vi "S4GUI.vi"(7 "Tab ObsEng":enum32{"Obs", "CCD modes", "Guider", "Eng"}(tab)) -> ()   [LabVIEW 2018] (continued)
      n64 = property on="Project ID" class="Str"(error in=w86, "Value"="" ("Observer"), "Text.BGColor"=u32 16448250) -> ()  [unwired: 1 in, 2 out]
      n65 = property on="SendExpose" class="Bool (strict)"(error in=w86, "Value"=TRUE ("ExtSync")) -> ()  [unwired: 1 in, 2 out]
      n66 = property on="suffix alert" class="Str"(error in=w86, "Text.BGColor"=u32 16711680, "Text.TextColor"=u32 16776722) -> ()  [unwired: 1 in, 2 out]
      n67 = property on="Object_dflat" class="Str"(error in=w86, "DisabledEnum"=w95) -> ()  [unwired: 1 in, 2 out]
      n68 = property on="Object_zero" class="Str"(error in=w86, "DisabledEnum"=w95) -> ()  [unwired: 1 in, 2 out]
      n69 = property on="Object_sflat" class="Str"(error in=w86, "DisabledEnum"=w95) -> ()  [unwired: 1 in, 2 out]
      n70 = local write "GUIDER"(FALSE ("GUIDER")) -> ()
      n71 = property on="Exptime ch1" class="DigNum (strict)"("Value"=w72) -> ()  [unwired: 2 in, 2 out]
      n72 = property on="Exptime ch2" class="DigNum (strict)"("Value"=w72) -> ()  [unwired: 2 in, 2 out]
      n73 = property on="Exptime ch3" class="DigNum (strict)"("Value"=w72) -> ()  [unwired: 2 in, 2 out]
      n74 = property on="Exptime ch4" class="DigNum (strict)"("Value"=w72) -> ()  [unwired: 2 in, 2 out]
      n75 = property on="dark suffix" class="Str"(error in=w82, "Text.BGColor"=u32 16448250) -> ()  [unwired: 1 in, 2 out]
      n76 = property on="object suffix" class="Str"(error in=w82, "Text.BGColor"=u32 16448250) -> (error out=w76:errorcluster)  [unwired: 1 in, 1 out]
      n77 = property on="dflat suffix" class="Str"(error in=w82, "Text.BGColor"=u32 16448250) -> ()  [unwired: 1 in, 2 out]
      n78 = property on="SET Temp message" class="Bool (strict)"(error in=w76, "Value"=TRUE ("SET Temp message")) -> (error out=w71:errorcluster)  [unwired: 1 in, 1 out]
      n79 = local write "TEST Comments"("Acquisition for testing purposes" ("TEST Comments")) -> ()
      n80 = local write "test suffix"("test" ("test suffix")) -> ()
      n81 = local write "Object_test"("TEST OBJECT" ("Object_test")) -> ()
      n82 = property on="sflat suffix" class="Str"(error in=w76, "Text.BGColor"=u32 16448250) -> ()  [unwired: 1 in, 2 out]
      n83 = property on="zero suffix" class="Str"(error in=w76, "Text.BGColor"=u32 16448250) -> ()  [unwired: 1 in, 2 out]
      n84 = property on="focus suffix" class="Str"(error in=w76, "Text.BGColor"=u32 16448250) -> ()  [unwired: 1 in, 2 out]
      "suffix alert" <- "Invalid char!" ("suffix alert")
      "FT warning" <- "" ("FT warning")
    }
    frame #4 {
      w97 = u32 1 ("# Cycles")
      n85 = local write "# Cycles"(w97) -> ()
      n86 = local write "#cycles ch1"(w97) -> ()
      n87 = local write "#cycles ch2"(w97) -> ()
      n88 = local write "#cycles ch3"(w97) -> ()
      n89 = local write "#cycles ch4"(w97) -> ()
      n90 = local write "Exp ch1"(w97) -> ()
      n91 = local write "Exp ch2"(w97) -> ()
      n92 = local write "Exp ch3"(w97) -> ()
      n93 = local write "Exp ch4"(w97) -> ()
    }
  }
  n94 = disable-structure shown="Enabled" {
    disable-tunnel: "S4ACS_GUI.lvclass" -> [w106 w108]
    disable-tunnel: w5 -> [w105 w107]
    disable-tunnel: [w100 w108] -> w25
    disable-tunnel: [w99 w107] -> w24
    frame Enabled {
      # "Carrega o ultimo filtro escolhido para os 4 canais."
      n95 = local read "Filter1"() -> (w104:u8)
      n96 = local read "Filter2"() -> (w103:u8)
      n97 = local read "Filter3"() -> (w102:u8)
      n98 = local read "Filter4"() -> (w101:u8)
      n99 = call-dynamic "LoadFilters.vi"("Filter 4"=w101, "Filter 3"=w102, "error in (no error)"=w105, "Filter 2"=w103, "Filter 1"=w104, "S4GUI in"=w106) -> ("error out"=w99:errorcluster, "S4GUI out"=w100:refnum<class "S4GUI.lvclass">)  [unwired: 4 in]
    }
    frame Disabled {
    }
  }
  n100 = flat-sequence "Indicadores dos canais da parte inferior da tela principal" {
    frame #0 {
      w109 = ""
      "B1" <- w109
      "PA1" <- w109
      "RO1" <- w109
      "G1" <- w109
      "SI2" <- w109
      "PA2" <- w109
      "G2" <- w109
      "B2" <- w109
      "RO2" <- w109
      "EA2" <- w109
      "SI3" <- w109
      "EA3" <- w109
      "PA3" <- w109
      "B3" <- w109
      "G3" <- w109
      "RO3" <- w109
      "SI4" <- w109
      "EA4" <- w109
      "PA4" <- w109
      "B4" <- w109
      "G4" <- w109
      "RO4" <- w109
      "SI1" <- w109
      "EA1" <- w109
    }
  }
  n101 = call-dynamic "Write GUI version.vi"("error in (no error)"=w24, "GUI version"=w22, "S4GUI in"=w25) -> ("error out"=w16:errorcluster, "S4GUI out"=w23:refnum<class "S4GUI.lvclass">)  [unwired: 7 in]
  n102 = property on="Tab Acq Type" class="TabCtl (strict)"(error in=w16, "DisabledEnum"=T12."Disabled and Grayed Out" ("Disabled")) -> (error out=w15:errorcluster)  [unwired: 1 in, 1 out]
  n103 = control-ref of="Current Configuration"() -> (w33:refnum<vi>)
  n104 = control-ref of="Parameters"() -> (w30:refnum<vi>)
  n105 = call-dynamic "Initialize.vi"("error in (no error)"=w15, "S4ACS_GUI in"=w23) -> ("error out"=w14:errorcluster, "S4ACS_GUI out"=w18:refnum<class "S4GUI.lvclass">)  [unwired: 8 in]
  n106 = property on="Tab Acq Type" class="TabCtl (strict)"(error in=w14, "DisabledEnum"=T12."Enabled" ("Disabled")) -> (error out=w13:errorcluster)  [unwired: 1 in, 1 out]
  n107 = property on="Property Node" class="Clust (strict)"(reference=w30, "Top"=230 ("Position:Top")) -> (reference out=w34:refnum<vi>)  [unwired: 1 in, 1 out]
  n108 = property on="Property Node" class="Clust (strict)"(reference=w33, "Top"=230 ("Position:Top")) -> (reference out=w32:refnum<vi>)  [unwired: 1 in, 1 out]
  n109 = call-dynamic "Read TabAcqType index.vi"("error in (no error)"=w13, "S4GUI in"=w18) -> ("error out"=w10:errorcluster, "TabAcqType index"=w17:u32, "S4GUI out"=w11:refnum<class "S4GUI.lvclass">)  [unwired: 7 in]
  n110 = case shown="1" w17 {
    tunnel: [T1."OBJECT" ("Tab Acq Type") T1."TEST" ("Tab Acq Type") T1."DFLAT" ("Tab Acq Type") T1."SFLAT" ("Tab Acq Type") T1."DARK" ("Tab Acq Type") T1."ZERO" ("Tab Acq Type") T1."FOCUS" ("Tab Acq Type")] -> w7
    frame 0, Default {
    }
    frame 1 {
    }
    frame 2 {
    }
    frame 3 {
    }
    frame 4 {
    }
    frame 5 {
    }
    frame 6 {
    }
  }
  n111 = local write "Tab Acq Type"(w7) -> ()
  n112 = Bundle("Parameters"=w34, "Current Configuration"=w32) -> (w31:T13)  [unwired: 1 in]
  n113 = call-dynamic "Write ExpMode.vi"("error in (no error)"=w10, "ExpMode"=w7, "S4GUI in"=w11) -> ("error out"=w9:errorcluster, "S4GUI out"=w8:refnum<class "S4GUI.lvclass">)  [unwired: 7 in]
  n114 = while {
    shift-right: [w135] -> w4
    shift-left: w8 -> [w137]
    shift-right: [w122] -> w2
    shift-left: w9 -> [w118]
    tunnel: w31 -> [w142]
    i -> [w128]
    stop <- w119 stop-if-true
    # "Sufixo do arquivo SEMPRE\nem minúsculas."
    n115 = case shown="\"TEST\"" "Tab Acq Type" {
      tunnel: ["object suffix" "test suffix" "dflat suffix" "sflat suffix" "dark suffix" "zero suffix" "focus suffix"] -> w130
      tunnel: ["OBJECT Comments" "TEST Comments" "DFLAT Comments" "SFLAT Comments" "DARK Comments" "ZERO Comments" "FOCUS Comments"] -> w143
      tunnel: ["OBJECT" "TEST" "FLAT" "FLAT" "DARK" "ZERO" "FOCUS"] -> w140
      tunnel: ["Object_obj" "Object_test" "DOMEFLAT" "SKYFLAT" "Object_dark" "ZERO" "Object_focus"] -> w139
      tunnel: [_ _ _ _ _ _ "Start focus"] -> w127
      tunnel: [_ _ _ _ _ _ "Step focus"] -> w125
      tunnel: [_ _ _ _ _ _ "#steps"] -> w126
      frame "OBJECT", Default {
      }
      frame "TEST" {
      }
      frame "DFLAT" {
      }
      frame "SFLAT" {
      }
      frame "DARK" {
      }
      frame "ZERO" {
      }
      frame "FOCUS" {
      }
    }
    n116 = flat-sequence {
      tunnel: w137 -> [w157]
      tunnel: [w157] -> w117
      tunnel: [w156] -> w134
      frame #0 {
        n117 = case shown="False" "reset max" {
          frame False {
          }
          frame True {
            n118 = local write "loop max(ms)"(u32 0 ("loop max(ms)")) -> ()
          }
        }
        n119 = Tick Count (ms)() -> (millisecond timer value=w156:u32)
      }
    }
    n120 = To Lower Case(string=w130) -> (all lower case string=w129:string)
    n121 = event shown="[44] \"Tab Acq Type\": Value Change" {
      selector: _ -> [_ _ _ _ _ _ _ _ _ _ _ _ _ _ _ _ _ _ _ _ _ _ _ _ _ _ _ _ _ _ _ _ _ _ _ _ _ _ _ _ _ _ _ _ _ _ _ _ _ _ _ _ _ _ _ _ _ _ _ _ _ _ _ _ _ _ _ _ _ _ _ _ _ _ _ _ _ _ _ _ _ _ _ _ _ _ _ _ _ _ _ _ _ _ _ _ _ _ _ _ _ _ _ _ _ _ _ _ _ _ _ _ _ _ _ _ _ _ _ _ _ _ _ _ _ _ _ _ _ _ _ _ _ _ _ _ _ _ _ _ _ _ _ _ _]
      dyn-events: _ -> [_ _ _ _ _ _ _ _ _ _ _ _ _ _ _ _ _ _ _ _ _ _ _ _ _ _ _ _ _ _ _ _ _ _ _ _ _ _ _ _ _ _ _ _ _ _ _ _ _ _ _ _ _ _ _ _ _ _ _ _ _ _ _ _ _ _ _ _ _ _ _ _ _ _ _ _ _ _ _ _ _ _ _ _ _ _ _ _ _ _ _ _ _ _ _ _ _ _ _ _ _ _ _ _ _ _ _ _ _ _ _ _ _ _ _ _ _ _ _ _ _ _ _ _ _ _ _ _ _ _ _ _ _ _ _ _ _ _ _ _ _ _ _ _ _]
      timeout: 20 -> [_ _ _ _ _ _ _ _ _ _ _ _ _ _ _ _ _ _ _ _ _ _ _ _ _ _ _ _ _ _ _ _ _ _ _ _ _ _ _ _ _ _ _ _ _ _ _ _ _ _ _ _ _ _ _ _ _ _ _ _ _ _ _ _ _ _ _ _ _ _ _ _ _ _ _ _ _ _ _ _ _ _ _ _ _ _ _ _ _ _ _ _ _ _ _ _ _ _ _ _ _ _ _ _ _ _ _ _ _ _ _ _ _ _ _ _ _ _ _ _ _ _ _ _ _ _ _ _ _ _ _ _ _ _ _ _ _ _ _ _ _ _ _ _ _]
      tunnel: w117 -> [w199 w2003 w2014 w2019 w2024 w2029 w2034 w2039 w2357 w2516 w2546 w2552 w2574 w2596 w2795 w2803 w2882 w2903 w2975 w3046 w3147 w3161 w3302 w3541 w3573 w3605 w3637 w3672 w3707 w3742 w3777 w3780 w3878 w4087 w4151 w4678 w4757 w4829 w4900 w4973 w5024 w5065 w5507 w5513 w5633 w7076 w7220 w7425 w7613 w7877 w8136 w8151 w8362 w8592 w8616 w8640 w8664 w8688 w8703 w8845 w8987 w9116 w9136 w9156 w9176 w9197 w9262 w9327 w9392 w9457 w9494 w9522 w9550 w9579 w9652 w9782 w9816 w9875 w9934 w9993 w10052 w10072 w10099 w10115 w10136 w10166 w10196 w10221 w10262 w10303 w10344 w10385 w10426 w10467 w10508 w10551 w10666 w10776 w10886 w10995 w11005 w11025 w11040 w11055 w11070 w11085 w11100 w11115 w11130 w11161 w11190 w11214 w11256 w11290 w11317 w11340 w11368 w11388 w11403 w11423 w11506 w11834 w11860 w12026 w12046 w12061 w12077 w12097 w12117 w12137 w12157 w12172 w12188 w12208 w12228 w12248 w12268 w12283 w12303 w12323 w12343 w12358 w12378 w12398 w12418]
      tunnel: w118 -> [w198 w2002 w2013 w2018 w2023 w2028 w2033 w2038 w2358 w2514 w2545 w2551 w2573 w2595 w2794 w2802 w2881 w2902 w2974 w3047 w3146 w3153 w3298 w3540 w3572 w3604 w3636 w3671 w3706 w3741 w3776 w3788 w3879 w4086 w4150 w4677 w4756 w4828 w4896 w4972 w5022 w5064 w5463 w5512 w5632 w7075 w7219 w7424 w7612 w7870 w8134 w8150 w8360 w8591 w8615 w8639 w8663 w8687 w8702 w8843 w8986 w9117 w9137 w9157 w9177 w9196 w9261 w9326 w9391 w9455 w9492 w9520 w9548 w9578 w9651 w9781 w9815 w9874 w9933 w9992 w10051 w10071 w10098 w10114 w10135 w10165 w10195 w10220 w10261 w10302 w10343 w10384 w10425 w10466 w10507 w10550 w10665 w10775 w10885 w10994 w11004 w11024 w11039 w11054 w11069 w11084 w11099 w11114 w11129 w11160 w11189 w11213 w11255 w11289 w11316 w11339 w11367 w11387 w11402 w11422 w11507 w11833 w11859 w12025 w12045 w12060 w12076 w12096 w12116 w12136 w12156 w12171 w12187 w12207 w12227 w12247 w12267 w12282 w12302 w12322 w12342 w12357 w12377 w12397 w12417]
      tunnel: [w195 w2001 w2011 w2015 w2020 w2025 w2030 w2035 w2320 w2508 w2533 w2553 w2575 w2597 w2782 w2820 w2881 w2920 w2992 w3064 w3133 w3159 w3300 w3451 w3559 w3591 w3623 w3662 w3697 w3732 w3767 w3788 w3801 w4007 w4138 w4597 w4754 w4826 w4891 w4970 w5025 w5059 w5466 w5509 w5600 w7129 w7213 w7418 w7624 w7871 w8135 w8143 w8348 w8522 w8598 w8623 w8647 w8671 w8689 w8832 w8972 w9115 w9135 w9155 w9175 w9195 w9260 w9325 w9390 w9456 w9493 w9521 w9549 w9583 w9656 w9783 w9814 w9873 w9932 w9991 w10050 w10070 w10097 w10113 w10134 w10164 w10194 w10223 w10264 w10305 w10346 w10387 w10428 w10469 w10510 w10549 w10664 w10774 w10884 w10991 w11003 w11023 w11038 w11053 w11068 w11083 w11098 w11113 w11128 w11145 w11187 w11212 w11254 w11288 w11315 w11338 w11350 w11370 w11390 w11406 w11430 w11841 w11864 w12008 w12028 w12048 w12069 w12082 w12102 w12119 w12139 w12159 w12176 w12191 w12211 w12230 w12250 w12270 w12286 w12305 w12325 w12345 w12361 w12380 w12400] -> w122
      tunnel: [w196 _ _ _ _ _ _ _ _ _ _ _ _ _ _ _ _ _ _ _ _ _ _ _ _ _ _ _ _ _ _ _ _ _ _ _ _ _ _ _ _ _ _ _ _ _ _ _ _ _ _ _ _ _ _ _ _ _ _ _ _ _ _ _ _ _ _ _ _ _ _ _ _ _ _ _ _ _ _ _ _ _ _ _ _ _ _ _ _ _ _ _ _ _ _ _ _ _ _ _ _ _ _ _ _ _ _ _ _ _ _ _ _ _ _ _ _ _ _ _ _ _ _ _ _ _ _ _ _ _ _ _ _ _ _ _ _ _ _ _ _ _ _ _ _] -> w120
      tunnel: w129 -> [_ _ _ _ _ _ _ _ _ _ _ _ _ _ _ _ _ _ _ _ _ _ _ _ _ _ _ _ _ _ _ _ _ _ _ _ _ _ _ _ _ w5058 _ _ _ _ w7218 w7422 _ w7875 _ w8148 w8369 _ _ _ _ _ w8710 w8852 w8994 _ _ _ _ _ _ _ _ _ _ _ _ _ _ _ _ _ _ _ _ _ _ _ _ _ _ _ _ _ _ _ _ _ _ _ _ _ _ _ _ _ _ _ _ _ _ _ _ _ _ _ _ _ _ _ _ _ _ _ _ _ _ _ _ _ _ _ _ _ _ _ _ _ _ _ _ _ _ _ _ _ _ _ _]
      tunnel: w143 -> [_ _ _ _ _ _ _ _ _ _ _ _ _ _ _ _ _ _ _ _ _ _ _ _ _ _ _ _ _ _ _ _ _ _ _ _ _ _ _ _ _ w5057 _ _ _ _ w7217 _ w7628 w7874 _ w8147 w8368 _ _ _ _ _ w8709 w8851 w8993 _ _ _ _ _ _ _ _ _ _ _ _ _ _ _ _ _ _ _ _ _ _ _ _ _ _ _ _ _ _ _ _ _ _ _ _ _ _ _ _ _ _ _ _ _ _ _ _ _ _ _ _ _ _ _ _ _ _ _ _ _ _ _ _ _ _ _ _ _ _ _ _ _ _ _ _ _ _ _ _ _ _ _ _]
      tunnel: w142 -> [_ _ _ _ _ _ _ _ _ _ _ _ _ _ _ _ _ _ _ _ _ _ _ _ _ _ _ _ _ _ _ w3781 _ _ _ _ _ _ _ _ _ _ _ _ _ _ _ _ _ _ _ _ _ _ _ _ _ _ _ _ _ _ _ _ _ _ _ _ _ _ _ _ _ _ _ _ _ _ _ _ _ _ _ _ _ _ _ _ _ _ _ _ _ _ _ _ _ _ _ _ _ _ _ _ _ _ _ _ _ _ _ _ _ _ _ _ _ _ _ _ _ _ _ _ _ _ _ _ _ _ _ _ _ _ _ _ _ _ _ _ _ _ _ _ _]
      tunnel: [w194 w2003 w2012 w2016 w2021 w2026 w2031 w2036 w2322 w2507 w2534 w2554 w2576 w2598 w2783 w2821 w2882 w2921 w2993 w3065 w3124 w3160 w3301 w3453 w3550 w3582 w3614 w3639 w3674 w3709 w3744 w3780 w3802 w4004 w4139 w4598 w4755 w4827 w4892 w4971 w5026 w5039 w5467 w5508 w5601 w7128 w7214 w7419 w7625 w7872 w8136 w8144 w8349 w8523 w8599 w8624 w8648 w8672 w8690 w8831 w8974 w9114 w9134 w9154 w9174 w9194 w9259 w9324 w9389 w9454 w9491 w9519 w9547 w9581 w9654 w9784 w9813 w9872 w9931 w9990 w10049 w10069 w10089 w10112 w10133 w10163 w10193 w10222 w10263 w10304 w10345 w10386 w10427 w10468 w10509 w10548 w10663 w10773 w10883 w10992 w10996 w11019 w11034 w11049 w11064 w11079 w11094 w11109 w11124 w11144 w11162 w11199 w11223 w11271 w11301 w11326 w11349 w11369 w11389 w11404 w11431 w11842 w11865 w12007 w12027 w12047 w12068 w12080 w12100 w12118 w12138 w12158 w12175 w12189 w12209 w12229 w12249 w12269 w12284 w12304 w12324 w12344 w12359 w12379 w12399] -> w136
      tunnel: "Input Cluster" -> [_ _ _ _ _ _ _ _ _ _ _ _ _ _ _ _ _ _ _ _ _ _ _ _ _ _ _ _ _ _ _ w3779 _ _ _ _ _ _ _ _ _ _ _ _ _ _ _ _ _ _ _ _ _ _ _ _ _ _ _ _ _ _ _ _ _ _ _ _ _ _ _ _ _ _ _ _ _ _ _ _ _ _ _ _ _ _ _ _ _ _ _ _ _ _ _ _ _ _ _ _ _ _ _ _ _ _ _ _ _ _ _ _ _ _ _ _ _ _ _ _ _ _ _ _ _ _ _ _ _ _ _ _ _ _ _ _ _ _ _ _ _ _ _ _ _]
      tunnel: w140 -> [_ _ _ _ _ _ _ _ _ _ _ _ _ _ _ _ _ _ _ _ _ _ _ _ _ _ _ _ _ _ _ _ _ _ _ _ _ _ _ _ _ w5056 _ _ _ _ w7215 w7420 w7626 w7873 _ w8145 w8367 _ _ _ _ _ w8708 w8849 w8992 _ _ _ _ _ _ _ _ _ _ _ _ _ _ _ _ _ _ _ _ _ _ _ _ _ _ _ _ _ _ _ _ _ _ _ _ _ _ _ _ _ _ _ _ _ _ _ _ _ _ _ _ _ _ _ _ _ _ _ _ _ _ _ _ _ _ _ _ _ _ _ _ _ _ _ _ _ _ _ _ _ _ _ _]
      tunnel: w139 -> [_ _ _ _ _ _ _ _ _ _ _ _ _ _ _ _ _ _ _ _ _ _ _ _ _ _ _ _ _ _ _ _ _ _ _ _ _ _ _ _ _ w5055 _ _ _ _ _ w7423 w7629 w7876 _ w8149 w8366 _ _ _ _ _ w8707 w8850 w8991 _ _ _ _ _ _ _ _ _ _ _ _ _ _ _ _ _ _ _ _ _ _ _ _ _ _ _ _ _ _ _ _ _ _ _ _ _ _ _ _ _ _ _ _ _ _ _ _ _ _ _ _ _ _ _ _ _ _ _ _ _ _ _ _ _ _ _ _ _ _ _ _ _ _ _ _ _ _ _ _ _ _ _ _]
      tunnel: "Observer" -> [_ _ _ _ _ _ _ _ _ _ _ _ _ _ _ _ _ _ _ _ _ _ _ _ _ _ _ _ _ _ _ _ _ _ _ _ _ _ _ _ _ w5054 _ _ w5606 w6963 w7216 w7421 w7627 _ _ w8146 w8365 _ _ _ _ _ w8706 w8848 w8990 _ _ _ _ _ _ _ _ _ _ _ _ _ _ _ _ _ _ _ _ _ _ _ _ _ _ _ _ _ _ _ _ _ _ _ _ _ _ _ _ _ _ _ _ _ _ _ _ _ _ _ _ _ _ _ _ _ _ _ _ _ _ _ _ _ _ _ _ _ _ _ _ _ _ _ _ _ _ _ _ _ _ _ _]
      tunnel: w128 -> [w197 _ _ _ _ _ _ _ _ _ _ _ _ _ _ _ _ _ _ _ _ _ _ _ _ _ _ _ _ _ _ _ _ _ _ _ _ _ _ _ _ _ _ _ _ _ _ _ _ _ _ _ _ _ _ _ _ _ _ _ _ _ _ _ _ _ _ _ _ _ _ _ _ _ _ _ _ _ _ _ _ _ _ _ _ _ _ _ _ _ _ _ _ _ _ _ _ _ _ _ _ _ _ _ _ _ _ _ _ _ _ _ _ _ _ _ _ _ _ _ _ _ _ _ _ _ _ _ _ _ _ _ _ _ _ _ _ _ _ _ _ _ _ _ _]
      tunnel: "Tab Acq Type" -> [_ _ _ _ _ _ _ _ _ _ _ _ _ _ _ _ _ _ _ _ _ _ _ _ _ _ _ _ _ _ _ _ _ _ _ _ _ _ _ _ _ w5046 _ _ _ _ _ _ w7615 _ _ _ w8356 _ _ _ _ _ w8697 w8839 w8980 _ _ _ _ _ _ _ _ _ _ _ _ _ _ _ _ _ _ _ _ _ _ _ _ _ _ _ _ _ _ _ _ _ _ _ _ _ _ _ _ _ _ _ _ _ _ _ _ _ _ _ _ _ _ _ _ _ _ _ _ _ _ _ _ _ _ _ _ _ _ _ _ _ _ _ _ _ _ _ _ _ _ _ _]
      tunnel: w127 -> [_ _ _ _ _ _ _ _ _ _ _ _ _ _ _ _ _ _ _ _ _ _ _ _ _ _ _ _ _ _ _ _ _ _ _ _ _ _ _ _ _ w5045 _ _ _ _ _ _ _ _ _ _ w8355 _ _ _ _ _ w8696 w8838 w8979 _ _ _ _ _ _ _ _ _ _ _ _ _ _ _ _ _ _ _ _ _ _ _ _ _ _ _ _ _ _ _ _ _ _ _ _ _ _ _ _ _ _ _ _ _ _ _ _ _ _ _ _ _ _ _ _ _ _ _ _ _ _ _ _ _ _ _ _ _ _ _ _ _ _ _ _ _ _ _ _ _ _ _ _]
      tunnel: w126 -> [_ _ _ _ _ _ _ _ _ _ _ _ _ _ _ _ _ _ _ _ _ _ _ _ _ _ _ _ _ _ _ _ _ _ _ _ _ _ _ _ _ w5043 _ _ _ _ _ _ _ _ _ _ w8353 _ _ _ _ _ w8694 w8836 w8977 _ _ _ _ _ _ _ _ _ _ _ _ _ _ _ _ _ _ _ _ _ _ _ _ _ _ _ _ _ _ _ _ _ _ _ _ _ _ _ _ _ _ _ _ _ _ _ _ _ _ _ _ _ _ _ _ _ _ _ _ _ _ _ _ _ _ _ _ _ _ _ _ _ _ _ _ _ _ _ _ _ _ _ _]
      tunnel: w125 -> [_ _ _ _ _ _ _ _ _ _ _ _ _ _ _ _ _ _ _ _ _ _ _ _ _ _ _ _ _ _ _ _ _ _ _ _ _ _ _ _ _ w5044 _ _ _ _ _ _ _ _ _ _ w8354 _ _ _ _ _ w8695 w8837 w8978 _ _ _ _ _ _ _ _ _ _ _ _ _ _ _ _ _ _ _ _ _ _ _ _ _ _ _ _ _ _ _ _ _ _ _ _ _ _ _ _ _ _ _ _ _ _ _ _ _ _ _ _ _ _ _ _ _ _ _ _ _ _ _ _ _ _ _ _ _ _ _ _ _ _ _ _ _ _ _ _ _ _ _ _]
      tunnel: "Project ID" -> [_ _ _ _ _ _ _ _ _ _ _ _ _ _ _ _ _ _ _ _ _ _ _ _ _ _ _ _ _ _ _ _ _ _ _ _ _ _ _ _ _ _ _ _ w5605 w6961 _ _ _ _ _ _ _ _ _ _ _ _ _ _ _ _ _ _ _ _ _ _ _ _ _ _ _ _ _ _ _ _ _ _ _ _ _ _ _ _ _ _ _ _ _ _ _ _ _ _ _ _ _ _ _ _ _ _ _ _ _ _ _ _ _ _ _ _ _ _ _ _ _ _ _ _ _ _ _ _ _ _ _ _ _ _ _ _ _ _ _ _ _ _ _ _ _ _ _]
      event Timeout {
        # "execução do botão\nOK do SET TEMP de\ntodos os canais."
        # "2024.07.02: Mostra as publicações das aplicações."
        # "Trata as tarefas para atender \naos clientes: Publisher"
        # "Conteudo dos indicadores"
        # "Status dos indicadores: Habilitado ou Desab."
        # "Obtém os valores de status dos\ndispositivos de cada servidor para\napresentar nos indicadores da GUI."
        # "Trata as tarefas individuais de \ncada servidor (ACS1,...,ACS4, \nICS, TCS, Focus,Weather)"
        # "Determina a sequência de\ntarefas dos servidores\npara uma observação, de \nacordo com o modo de \noperação (disparado com \nos botões START)"
        # "execução dos botões\n no modo sincrono."
        # "execução dos botões\n no modo assincrono."
        n122 = event-data() -> ()  [unwired: 1 in, 2 out]
        n123 = disable-structure shown="Enabled" {
          disable-tunnel: w199 -> [w236 _]
          disable-tunnel: w198 -> [w234 _]
          frame Disabled {
            n124 = flat-sequence {
              tunnel: [w245] -> w235
              tunnel: w236 -> [w245]
              tunnel: w234 -> [w244]
              tunnel: [w244] -> w233
              frame #0 {
                n125 = local read "time alert"() -> (w242:u32)
                n126 = Tick Count (ms)() -> (millisecond timer value=w243:u32)
                n127 = Subtract(x=w243, y=w242) -> (x-y=w241:u32)
                n128 = Greater?(x=w241, y=u32 750) -> (0:w239:bool)
                n129 = case shown="True" w239 {
                  frame False {
                  }
                  frame True {
                    n130 = property on="suffix alert" class="Str"("Visible"=FALSE) -> ()  [unwired: 2 in, 2 out]
                  }
                }
              }
            }
            n131 = local read "charKeyboardInteger"() -> (w237:i16)
            n132 = call-dynamic "Read ExpMode.vi"("error in (no error)"=w233, "S4GUI in"=w235) -> ("ExpMode"=w238:T1)  [unwired: 7 in, 2 out]
            n133 = case shown="Default" w237 {
              tunnel: w238 -> [_ w247 w269]
              frame 32767 {
              }
              frame 0, 8, 32, 48..57, 65..90, 97..122 {
                n134 = case shown="\"OBJECT\", Default" w247 {
                  tunnel: [w252 w253 w254 w255 w256 w257] -> w248
                  frame "OBJECT", Default {
                    n135 = local read "object suffix"() -> (w252:string)
                  }
                  frame "DFLAT" {
                    n136 = local read "dflat suffix"() -> (w253:string)
                  }
                  frame "SFLAT" {
                    n137 = local read "sflat suffix"() -> (w254:string)
                  }
                  frame "DARK" {
                    n138 = local read "dark suffix"() -> (w255:string)
                  }
                  frame "ZERO" {
                    n139 = local read "zero suffix"() -> (w256:string)
                  }
                  frame "FOCUS" {
                    n140 = local read "focus suffix"() -> (w257:string)
                  }
                }
                n141 = String Length(string=w248) -> (length=w251:i32)
                n142 = Greater?(x=w251, y=10) -> (0:w249:bool)
                n143 = case shown="True" w249 {
                  tunnel: w248 -> [w258 _]
                  tunnel: w247 -> [_ w260]
                  frame False {
                    n144 = local write "suffix temp"(w258) -> ()
                  }
                  frame True {
                    n145 = local read "suffix temp"() -> (w259:string)
                    n146 = case shown="\"OBJECT\", Default" w260 {
                      tunnel: w259 -> [w261 w262 w263 w264 w265 w266]
                      frame "OBJECT", Default {
                        n147 = local write "object suffix"(w261) -> ()
                      }
                      frame "DFLAT" {
                        n148 = local write "dflat suffix"(w262) -> ()
                      }
                      frame "SFLAT" {
                        n149 = local write "sflat suffix"(w263) -> ()
                      }
                      frame "DARK" {
                        n150 = local write "dark suffix"(w264) -> ()
                      }
                      frame "ZERO" {
                        n151 = local write "zero suffix"(w265) -> ()
                      }
                      frame "FOCUS" {
                        n152 = local write "focus suffix"(w266) -> ()
                      }
                    }
                  }
                }
              }
              frame Default {
                n153 = local write "charKeyboardInteger"(i16 32767 ("lastChar")) -> ()
                n154 = Tick Count (ms)() -> (millisecond timer value=→"time alert":u32)
                n155 = property on="suffix alert" class="Str"("Visible"=TRUE) -> ()  [unwired: 2 in, 2 out]
                n156 = case shown="\"OBJECT\", Default" w269 {
                  tunnel: "suffix temp" -> [w272 w273 w274 w275 w276 w277]
                  frame "OBJECT", Default {
                    n157 = local write "object suffix"(w272) -> ()
                  }
                  frame "DFLAT" {
                    n158 = local write "dflat suffix"(w273) -> ()
                  }
                  frame "SFLAT" {
                    n159 = local write "sflat suffix"(w274) -> ()
                  }
                  frame "DARK" {
                    n160 = local write "dark suffix"(w275) -> ()
                  }
                  frame "ZERO" {
                    n161 = local write "zero suffix"(w276) -> ()
                  }
                  frame "FOCUS" {
                    n162 = local write "focus suffix"(w277) -> ()
                  }
                }
              }
            }
          }
          frame Enabled {
          }
        }
        n163 = disable-structure shown="Enabled" {
          disable-tunnel: w199 -> [w283 w288]
          disable-tunnel: w198 -> [w282 w286]
          disable-tunnel: [w280 w285] -> w191
          disable-tunnel: [w279 w284] -> w193
          disable-tunnel: w197 -> [_ w287]
          frame Disabled {
            n164 = call "Elapsed Time"() -> ("Time has Elapsed"=w278:bool)  [unwired: 12 in, 7 out]
            n165 = call "Elapsed Time3"() -> ("Time has Elapsed"=w281:bool)  [unwired: 12 in, 7 out]
            n166 = call "Write Status_timeout.vi"("error in (no error)"=w282, "TCS_timeout"=w281, "Status_timeout"=w278, "S4ACS_GUI in"=w283) -> ("error out"=w280:errorcluster, "S4ACS_GUI out"=w279:refnum<class "S4GUI.lvclass">)  [unwired: 6 in]
          }
          frame Enabled {
            n167 = call-dynamic "Write loop counter.vi"("error in (no error)"=w286, "loop counter"=w287, "S4GUI in"=w288) -> ("error out"=w285:errorcluster, "S4GUI out"=w284:refnum<class "S4GUI.lvclass">)  [unwired: 7 in]
          }
        }
        n168 = call-dynamic "HandleSetTemp.vi"("error in (no error)"=w191, "S4GUI in"=w193) -> ("error out"=w190:errorcluster, "S4GUI out"=w192:refnum<class "S4GUI.lvclass">)  [unwired: 8 in]
        n169 = call-dynamic "GetPubs.vi"("error in (no error)"=w190, "S4GUI in"=w192) -> ("error out"=w210:errorcluster, "Pubs out"=→"All Pubs":T11, "S4GUI out"=w209:refnum<class "S4GUI.lvclass">)  [unwired: 7 in]
        n170 = call-dynamic "HandlePauseAsync.vi"("error in (no error)"=w210, "S4GUI in"=w209) -> ("error out"=w227:errorcluster, "S4GUI out"=w229:refnum<class "S4GUI.lvclass">)  [unwired: 8 in]
        n171 = call-dynamic "HandleStopAsync.vi"("error in (no error)"=w227, "S4GUI in"=w229) -> ("error out"=w226:errorcluster, "S4GUI out"=w228:refnum<class "S4GUI.lvclass">)  [unwired: 8 in]
        n172 = call-dynamic "HandleAbortAsync.vi"("error in (no error)"=w226, "S4GUI in"=w228) -> ("error out"=w220:errorcluster, "S4GUI out"=w221:refnum<class "S4GUI.lvclass">)  [unwired: 8 in]
        n173 = call-dynamic "HandlePauseSync.vi"("error in (no error)"=w220, "S4GUI in"=w221) -> ("error out"=w219:errorcluster, "S4GUI out"=w218:refnum<class "S4GUI.lvclass">)  [unwired: 8 in]
        n174 = call-dynamic "HandleStopSync.vi"("error in (no error)"=w219, "S4GUI in"=w218) -> ("error out"=w223:errorcluster, "S4GUI out"=w225:refnum<class "S4GUI.lvclass">)  [unwired: 8 in]
        n175 = call-dynamic "HandleAbortSync.vi"("error in (no error)"=w223, "S4GUI in"=w225) -> ("error out"=w222:errorcluster, "S4GUI out"=w224:refnum<class "S4GUI.lvclass">)  [unwired: 8 in]
        n176 = call-dynamic "HandleObservation.vi"("error in (no error)"=w222, "S4ACS_GUI in"=w224) -> ("error out"=w231:errorcluster, "S4ACS_GUI out"=w232:refnum<class "S4GUI.lvclass">)  [unwired: 8 in]
        n177 = call-dynamic "HandleServers.vi"("error in (no error)"=w231, "S4GUI in"=w232) -> ("error out"=w213:errorcluster, "S4GUI out"=w214:refnum<class "S4GUI.lvclass">)  [unwired: 8 in]
        n178 = call-dynamic "HandleClients.vi"("error in (no error)"=w213, "S4GUI in"=w214) -> ("error out"=w212:errorcluster, "S4GUI out"=w204:refnum<class "S4GUI.lvclass">)  [unwired: 8 in]
        n179 = call-dynamic "GetStatus.vi"("error in (no error)"=w212, "S4GUI in"=w204) -> ("error out"=w206:errorcluster, "S4GUI out"=w203:refnum<class "S4GUI.lvclass">)  [unwired: 8 in]
        n180 = call-dynamic "Read output cluster.vi"("error in (no error)"=w206, "S4GUI in"=w203) -> ("error out"=w205:errorcluster, "output cluster"=w200:T15, "S4GUI out"=w202:refnum<class "S4GUI.lvclass">)  [unwired: 7 in]
        n181 = call "Elapsed Time2"() -> ("Time has Elapsed"=w217:bool)  [unwired: 12 in, 7 out]
        n182 = call-dynamic "Read Cluster Disable.vi"("error in (no error)"=w205, "S4GUI in"=w202) -> ("error out"=w207:errorcluster, "Cluster Disable"=w208:T16, "S4GUI out"=w201:refnum<class "S4GUI.lvclass">)  [unwired: 7 in]
        n183 = call "Read cfg file.vi"("error in (no error)"=w207, "S4ACS_GUI in"=w201) -> ("error out"=w215:errorcluster, "cfg file"=w230:string, "S4ACS_GUI out"=w216:refnum<class "S4GUI.lvclass">)  [unwired: 7 in]
        n184 = case shown="True" w217 {
          tunnel: w200 -> [_ w346]
          tunnel: w208 -> [_ w345]
          tunnel: w230 -> [_ w344]
          tunnel: w216 -> [w291 w343]
          tunnel: w215 -> [w290 w342]
          tunnel: [w290 w295] -> w195
          tunnel: [FALSE ("exit") w294] -> w196
          tunnel: [w291 w293] -> w194
          frame False {
          }
          frame True {
            w302 = "arking" ("regular expression")
            w320 = "ERRO" ("regular expression")
            # "Verifica mudança de modo e se deve carregar valores default \npara procedimento de ajuste de foco do telescópio."
            # "1a vez FOTOM (F)"
            # "1a vez POLAR (F)"
            # "MODE:\nF -> photometric\nT -> polarimetric"
            n185 = stacked-sequence {
              tunnel: w343 -> [w395 w402 w413 w423 w432]
              tunnel: w342 -> [w394 w401 w412 w422 w431]
              tunnel: [_ _ _ _ w430] -> w336
              tunnel: [_ _ _ _ w429] -> w335
              tunnel: [_ _ _ _ w428] -> w305
              frame #0 {
                n186 = call-dynamic "Read AcquisitionA.vi"("error in (no error)"=w394, "S4ACS_GUI in"=w395) -> ("error out"=w391:errorcluster, "Acquisition.lvclass"=w393:refnum<class "Acquisition.lvclass">)  [unwired: 7 in, 1 out]
                n187 = call-dynamic "Read Channel.vi"("error in (no error)"=w391, "Acquisition in"=w393) -> ("error out"=w390:errorcluster, "Channel.lvclass"=w392:refnum<class "Channel.lvclass">)  [unwired: 7 in, 1 out]
                n188 = call-dynamic "Read CyclesDone.vi"("error in (no error)"=w390, "Channel in"=w392) -> ("error out"=→"error out 6":errorcluster, "CyclesDone"=w387:u32)  [unwired: 7 in, 1 out]
                "Cycles Done ch1" <- w387
                n189 = Number To Decimal String(number=w387) -> (decimal integer string=w386:string)  [unwired: 1 in]
                n190 = Concatenate Strings("#Cycles Done ", w386) -> (w385:string)
                n191 = property on="Cycles Done ch1" class="Slide (strict)"("Caption.Text"=w385) -> ()  [unwired: 2 in, 2 out]
              }
              frame #1 {
                n192 = call "Read AcquisitionB.vi"("error in (no error)"=w401, "S4ACS_GUI in"=w402) -> ("error out"=w404:errorcluster, "Acquisition.lvclass"=w405:refnum<class "Acquisition.lvclass">)  [unwired: 7 in, 1 out]
                n193 = call-dynamic "Read Channel.vi"("error in (no error)"=w404, "Acquisition in"=w405) -> ("error out"=w403:errorcluster, "Channel.lvclass"=w406:refnum<class "Channel.lvclass">)  [unwired: 7 in, 1 out]
                n194 = call-dynamic "Read CyclesDone.vi"("error in (no error)"=w403, "Channel in"=w406) -> ("error out"=→"error out 4":errorcluster, "CyclesDone"=w397:u32)  [unwired: 7 in, 1 out]
                "Cycles Done ch2" <- w397
                n195 = Number To Decimal String(number=w397) -> (decimal integer string=w398:string)  [unwired: 1 in]
                n196 = Concatenate Strings("#Cycles Done ", w398) -> (w396:string)
                n197 = property on="Cycles Done ch2" class="Slide (strict)"("Caption.Text"=w396) -> ()  [unwired: 2 in, 2 out]
              }
              frame #2 {
                n198 = call-dynamic "Read AcquisitionC.vi"("error in (no error)"=w412, "S4ACS_GUI in"=w413) -> ("error out"=w415:errorcluster, "Acquisition.lvclass"=w416:refnum<class "Acquisition.lvclass">)  [unwired: 7 in, 1 out]
                n199 = call-dynamic "Read Channel.vi"("error in (no error)"=w415, "Acquisition in"=w416) -> ("error out"=w414:errorcluster, "Channel.lvclass"=w417:refnum<class "Channel.lvclass">)  [unwired: 7 in, 1 out]
                n200 = call-dynamic "Read CyclesDone.vi"("error in (no error)"=w414, "Channel in"=w417) -> ("error out"=→"error out 5":errorcluster, "CyclesDone"=w408:u32)  [unwired: 7 in, 1 out]
                "Cycles Done ch3" <- w408
                n201 = Number To Decimal String(number=w408) -> (decimal integer string=w409:string)  [unwired: 1 in]
                n202 = Concatenate Strings("#Cycles Done ", w409) -> (w407:string)
                n203 = property on="Cycles Done ch3" class="Slide (strict)"("Caption.Text"=w407) -> ()  [unwired: 2 in, 2 out]
              }
              frame #3 {
                n204 = call-dynamic "Read AcquisitionD.vi"("error in (no error)"=w422, "S4ACS_GUI in"=w423) -> ("error out"=w425:errorcluster, "Acquisition.lvclass"=w426:refnum<class "Acquisition.lvclass">)  [unwired: 7 in, 1 out]
                n205 = call-dynamic "Read Channel.vi"("error in (no error)"=w425, "Acquisition in"=w426) -> ("error out"=w424:errorcluster, "Channel.lvclass"=w427:refnum<class "Channel.lvclass">)  [unwired: 7 in, 1 out]
                n206 = call-dynamic "Read CyclesDone.vi"("error in (no error)"=w424, "Channel in"=w427) -> ("CyclesDone"=w419:u32)  [unwired: 7 in, 2 out]
                "Cycles Done ch4" <- w419
                n207 = Number To Decimal String(number=w419) -> (decimal integer string=w420:string)  [unwired: 1 in]
                n208 = Concatenate Strings("#Cycles Done ", w420) -> (w418:string)
                n209 = property on="Cycles Done ch4" class="Slide (strict)"("Caption.Text"=w418) -> ()  [unwired: 2 in, 2 out]
              }
              frame #4 {
                n210 = call-dynamic "Read SET request.vi"("error in (no error)"=w431, "S4GUI in"=w432) -> ("error out"=w429:errorcluster, "SET request"=w428:bool, "S4GUI out"=w430:refnum<class "S4GUI.lvclass">)  [unwired: 7 in]
              }
            }
            n211 = call-dynamic "Read Obs_state.vi"("error in (no error)"=w335, "S4ACS_GUI in"=w336) -> ("error out"=w313:errorcluster, "Obs_state"=w292:u32, "S4ACS_GUI out"=w314:refnum<class "S4GUI.lvclass">)  [unwired: 7 in]
            n212 = stacked-sequence {
              tunnel: w346 -> [w478 w488 w500 w502 w510 w556 w559 w693 w799 w1142 _ _ _ _ _ w1338 w1524 w1687 w1846 w1956]
              tunnel: [_ _ _ _ _ _ _ w691 _ _ _ _ _ _ _ _ _ _ _ _] -> w327
              tunnel: w345 -> [_ w484 _ _ _ _ _ _ _ _ w1173 w1220 w1237 w1254 w1271 _ _ _ _ _]
              tunnel: w344 -> [_ _ _ _ _ _ _ _ _ _ _ _ _ _ _ w1333 _ _ _ _]
              tunnel: w305 -> [_ _ _ _ _ _ _ _ _ _ _ _ _ _ _ _ _ _ _ w1959]
              tunnel: w292 -> [_ _ _ _ _ _ _ _ _ w1136 _ _ _ _ _ _ _ _ _ _]
              frame #0 {
                (unwired) u32 240 ("Tab Control Pane Dimension:Width")
                (unwired) u32 300 ("Tab Control Pane Dimension:Height")
                n213 = Unbundle By Name(w478) -> ("GS STATUS cluster.AG"=→"GUIDER":bool, "TCS id"=w444:u32, "TCSPD_connection"=→"TCSPD":bool, "TCS extended"=w475:string, "focus pos"=w440:i32, "weather status"=w438:T17)
                n214 = Unbundle By Name(w438) -> ("outTemp"=→"Outside Temp":string, "pressure"=→"Pressure":string, "outHumidity"=→"Humidity":string, "windSpeed"=→"Wind Speed[Km/h]":string)
                n215 = Number To Decimal String(number=w440) -> (decimal integer string=→"Telescope Focus":string)  [unwired: 1 in]
                n216 = Equal?(x=u32 6 ("Tab Control Pane Dimension:Width"), y=w444) -> (x = y?=w443:bool)
                n217 = Match Pattern(string=w475, regular expression="RA=") -> (after substring=w471:string)  [unwired: 1 in, 3 out]
                n218 = local write "TCS mode"(w443) -> ()
                n219 = Match Pattern(string=w471, regular expression="DEC=") -> (before substring=→"RA":string, after substring=w470:string)  [unwired: 1 in, 2 out]
                n220 = Match Pattern(string=w470, regular expression="EQUINOX=") -> (before substring=→"DEC":string, after substring=w469:string)  [unwired: 1 in, 2 out]
                n221 = Match Pattern(string=w469, regular expression="AIRMASS=") -> (after substring=w465:string)  [unwired: 1 in, 3 out]
                n222 = Match Pattern(string=w465, regular expression="TCSHA=") -> (before substring=→"Air Mass":string, after substring=w464:string)  [unwired: 1 in, 2 out]
                n223 = Match Pattern(string=w464, regular expression="TCSDATE=") -> (before substring=→"Hour Angle":string, after substring=w462:string)  [unwired: 1 in, 2 out]
                n224 = Match Pattern(string=w462, regular expression="TELFOCUS=") -> (before substring=→"Date":string, after substring=w458:string)  [unwired: 1 in, 2 out]
                n225 = Match Pattern(string=w458, regular expression="EXTTEMP=") -> (after substring=w457:string)  [unwired: 1 in, 3 out]
                n226 = Match Pattern(string=w457, regular expression="PRESSURE=") -> (after substring=w456:string)  [unwired: 1 in, 3 out]
                n227 = Match Pattern(string=w456, regular expression="HUMIDITY=") -> (after substring=w448:string)  [unwired: 1 in, 3 out]
                n228 = Match Pattern(string=w448, regular expression="JD=") -> (after substring=w449:string)  [unwired: 1 in, 3 out]
                n229 = disable-structure shown="Enabled" {
                  disable-tunnel: u32 211 ("Tab Control Pane Dimension:Height") -> [w480 _]
                  disable-tunnel: u32 225 ("Tab Control Pane Dimension:Width") -> [w479 _]
                  frame Disabled {
                    n230 = property on="Tab CH1" class="TabCtl (strict)"("PaneHeight"=w480, "PaneWidth"=w479) -> ()  [unwired: 2 in, 2 out]
                    n231 = property on="Tab CH2" class="TabCtl (strict)"("PaneHeight"=w480, "PaneWidth"=w479) -> ()  [unwired: 2 in, 2 out]
                    n232 = property on="Tab CH3" class="TabCtl (strict)"("PaneHeight"=w480, "PaneWidth"=w479) -> ()  [unwired: 2 in, 2 out]
                    n233 = property on="Tab CH4" class="TabCtl (strict)"("PaneHeight"=w480, "PaneWidth"=w479) -> ()  [unwired: 2 in, 2 out]
                  }
                  frame Enabled {
                  }
                }
                n234 = Match Pattern(string=w449, regular expression="SD=") -> (before substring=→"Julian Date":string, after substring=→"Sideral Time":string)  [unwired: 1 in, 2 out]
              }
              frame #1 {
                # "OV 2024 09 04: Depois da criação da aba CCD modes, TODOS os parametros da aba Camera são protegidos por senha, \ninclusive as chaves de habilitação dos canais."
                n235 = Unbundle By Name(w488) -> ("S4ICS id"=w486:u32)
                n236 = Unbundle By Name(w484) -> ("Cluster AdmCCDsetup.param"=w481:T12)
                n237 = Equal?(x=u32 11, y=w486) -> (x = y?=w485:bool)
                n238 = local write "S4ICS protocol"(w485) -> ()
                n239 = case shown="\"Disabled and Grayed Out\"" w481 {
                  tunnel: [_ w490 w494] -> w483
                  frame Default {
                  }
                  frame "Disabled" {
                    n240 = Build Array(u32 4 ("element"), u32 5 ("element"), u32 6 ("element")) -> (w490:u32[])
                  }
                  frame "Disabled and Grayed Out" {
                    n241 = Build Array(u32 4 ("element"), u32 5 ("element"), u32 6 ("element")) -> (w494:u32[])
                  }
                }
                n242 = property on="Trigger\nMode" class="Ring (strict)"("DisabledEnum"=w481) -> ()  [unwired: 2 in, 2 out]
                n243 = property on="Vertical\nShift Speed" class="Ring (strict)"("DisabledEnum"=w481) -> ()  [unwired: 2 in, 2 out]
                n244 = property on="Vertical\nClock Voltage" class="Ring (strict)"("DisabledEnum"=w481) -> ()  [unwired: 2 in, 2 out]
                n245 = To Long Integer(number=w483) -> (32bit integer=w482:i32[])
                n246 = property on="EM Gain" class="DigNum (strict)"("DisabledEnum"=w481) -> ()  [unwired: 2 in, 2 out]
                n247 = property on="Read\nMode" class="Ring (strict)"("DisabledEnum"=w481) -> ()  [unwired: 2 in, 2 out]
                n248 = property on="AQM" class="Enum (strict)"("Disabled Items []"=w482) -> ()  [unwired: 2 in, 2 out]
                n249 = property on="Acquisition\nMode" class="Ring (strict)"("DisabledEnum"=w481) -> ()  [unwired: 2 in, 2 out]
                n250 = property on="A/D \nChannel" class="DigNum (strict)"("DisabledEnum"=w481) -> ()  [unwired: 2 in, 2 out]
                n251 = property on="Readout\nRate" class="Ring (strict)"("DisabledEnum"=w481) -> ()  [unwired: 2 in, 2 out]
                n252 = property on="CCD \nEM Mode" class="Ring (strict)"("DisabledEnum"=w481) -> ()  [unwired: 2 in, 2 out]
                n253 = property on="CCD\nEM Gain" class="DigNum (strict)"("DisabledEnum"=w481) -> ()  [unwired: 2 in, 2 out]
                n254 = property on="Shutter\nTTL" class="Ring (strict)"("DisabledEnum"=w481) -> ()  [unwired: 2 in, 2 out]
                n255 = property on="Shutter\nOpenning Time" class="DigNum (strict)"("DisabledEnum"=w481) -> ()  [unwired: 2 in, 2 out]
                n256 = property on="Frame\nTransfer" class="Bool (strict)"("DisabledEnum"=w481) -> ()  [unwired: 2 in, 2 out]
                n257 = property on="Shutter\nMode" class="Ring (strict)"("DisabledEnum"=w481) -> ()  [unwired: 2 in, 2 out]
                n258 = property on="Pre-amplification\nGain" class="Ring (strict)"("DisabledEnum"=w481) -> ()  [unwired: 2 in, 2 out]
                n259 = property on="Shutter\nClosing Time" class="DigNum (strict)"("DisabledEnum"=w481) -> ()  [unwired: 2 in, 2 out]
                n260 = property on="Horizontal\nBinning" class="DigNum (strict)"("DisabledEnum"=w481) -> ()  [unwired: 2 in, 2 out]
                n261 = property on="Vertical\nBinning" class="DigNum (strict)"("DisabledEnum"=w481) -> ()  [unwired: 2 in, 2 out]
                n262 = property on="Image\nFInal Column" class="DigNum (strict)"("DisabledEnum"=w481) -> ()  [unwired: 2 in, 2 out]
                n263 = property on="CH1on" class="Bool (strict)"("DisabledEnum"=w481) -> ()  [unwired: 2 in, 2 out]
                n264 = property on="CH2on" class="Bool (strict)"("DisabledEnum"=w481) -> ()  [unwired: 2 in, 2 out]
                n265 = property on="CH3 on" class="Bool (strict)"("DisabledEnum"=w481) -> ()  [unwired: 2 in, 2 out]
                n266 = property on="CH4 on" class="Bool (strict)"("DisabledEnum"=w481) -> ()  [unwired: 2 in, 2 out]
                n267 = property on="Image\nFinal Line" class="DigNum (strict)"("DisabledEnum"=w481) -> ()  [unwired: 2 in, 2 out]
                n268 = property on="Image\nInitial Column" class="DigNum (strict)"("DisabledEnum"=w481) -> ()  [unwired: 2 in, 2 out]
                n269 = property on="Image \nInitial Line" class="DigNum (strict)"("DisabledEnum"=w481) -> ()  [unwired: 2 in, 2 out]
              }
              frame #2 {
                n270 = Unbundle By Name(w500) -> ("Trigger Mode Status"=→"String":string, "Focus_connection"=→"Focus 160":bool, "WS_connection"=→"Weather":bool)
              }
              frame #3 {
                n271 = Unbundle By Name(w502) -> ("Trigger General Status"=→"String 2":string)
              }
              frame #4 {
                n272 = Unbundle By Name(w510) -> ("Instrument Motor error"=w503:T18, "Instrument Status"=w504:T19, "Instrument States.WPROT State"=w509:i32, "Instrument Pos Names.WPROT posname"=w508:string, "Instrument Pos Names.WPSEL posname"=w507:string, "Instrument Pos Names.CALW posname"=w506:string, "Instrument Pos Names.ASEL posname"=w505:string)
                n273 = stacked-sequence {
                  tunnel: w504 -> [w517 w522 w527 w531 w535 w540 w545 w551 w553]
                  tunnel: w509 -> [w513 _ _ _ _ _ _ _ _]
                  tunnel: w508 -> [_ w520 _ _ _ _ _ _ _]
                  tunnel: w507 -> [_ _ w525 _ _ _ _ _ _]
                  tunnel: w506 -> [_ _ _ _ _ w538 _ _ _]
                  tunnel: w505 -> [_ _ _ _ _ _ w543 _ _]
                  tunnel: w503 -> [_ w519 w524 w530 w534 w537 w542 _ _]
                  frame #0 {
                    # "Pisca quando BUSY"
                    n274 = Unbundle By Name(w517) -> ("WPROT pos"=w514:dbl)
                    "WaveplatePos 2" <- w514
                    n275 = Equal?(x=w513, y=3) -> (x = y?=w511:bool)
                    n276 = property on="WaveplatePos 2" class="DigNum (strict)"("Blinking"=w511) -> ()  [unwired: 2 in, 2 out]
                    n277 = Number To Fractional String(number=w514, precision (6)=i16 1) -> (F-format string=→"Angle":string)  [unwired: 2 in]
                  }
                  frame #1 {
                    n278 = Unbundle By Name(w519) -> ("WPROT error"=→"WPROT motor error":bool)
                    n279 = Unbundle By Name(w522) -> ("WPROT pos"=→"Position WPROT":dbl)
                    "PosName WPROT" <- w520
                  }
                  frame #2 {
                    n280 = Unbundle By Name(w527) -> ("WPSEL pos"=→"Position WPSEL":dbl)
                    n281 = Unbundle By Name(w524) -> ("WPSEL error"=→"WPSEL motor error":bool)
                    "PosName WPSEL" <- w525
                  }
                  frame #3 {
                    n282 = Unbundle By Name(w531) -> ("GMIR pos"=→"Position GMIR" →"Position GMIR 2":dbl)
                    n283 = Unbundle By Name(w530) -> ("GMIR error"=→"GMIR motor error" →"GMIR motor error 2":bool)
                  }
                  frame #4 {
                    n284 = Unbundle By Name(w535) -> ("GFOC pos"=→"Position GFOC" →"Position GFOC 2":dbl)
                    n285 = Unbundle By Name(w534) -> ("GFOC error"=→"GFOC motor error" →"GFOC motor error 2":bool)
                  }
                  frame #5 {
                    n286 = Unbundle By Name(w540) -> ("CALW pos"=→"Position CALW":dbl)
                    n287 = Unbundle By Name(w537) -> ("CALW error"=→"CALW motor error":bool)
                    "PosName CALW" <- w538
                  }
                  frame #6 {
                    n288 = Unbundle By Name(w545) -> ("ASEL pos"=→"PosName ASEL":dbl)
                    n289 = Unbundle By Name(w542) -> ("ASEL error"=→"ASEL motor error":bool)
                    "PosName ASEL" <- w543
                  }
                  frame #7 {
                    w547 = cluster{u32, u32}[] [{16711680, 16711680}, {15400704, 15400704}, {16776722, 0}, {16776722, 0}]  # amarelo
                    w546 = cluster{u32, u32}[] [{16711680, 16711680}, {6618880, 6618880}, {16776722, 0}, {16776722, 0}]  # verde
                    n290 = Unbundle By Name(w551) -> ("connection"=→"S4ICSoft":bool, "operational"=w549:bool)
                    n291 = Select(t=w546, s=w549, f=w547) -> (s? t:f=w548:cluster{u32, u32}[])
                    n292 = property on="S4ICSoft" class="Bool (strict)"("Colors [4]"=w548) -> ()  [unwired: 2 in, 2 out]
                  }
                  frame #8 {
                    n293 = Unbundle By Name(w553) -> ("String Status"=→"Status":string)
                  }
                }
              }
              frame #5 {
                n294 = Unbundle By Name(w556) -> ("Sync Box State"=→"Current State":i32, "Trigger_connection"=→"Sync Box" →"LedExtSync":bool)
              }
              frame #6 {
                # "Instrument States.<device> State\n\n0: nao fez INIT e está parado (mode = IDLE ou WAITING\n                                                    contdition = default)\n1: nao fez INIT e está movendo (mode = IDLE ou WAITING\n                                                    contdition = BUSY)\n\n2: fez INIT e está parado (mode = default)\n                                            condition = READY)\n3: fez INIT e está movendo (mode = default)\n                                            condition = BUSY)"
                n295 = Unbundle By Name(w559) -> ("Instrument States"=w558:T20, "Instrument Pos Names"=w557:T21)
                n296 = stacked-sequence {
                  tunnel: w558 -> [w567 w589 w607 w641 w670]
                  tunnel: w557 -> [w563 _ w605 w637 _]
                  frame #0 {
                    # "WPSEL"
                    n297 = Unbundle By Name(w563) -> ("WPSEL posname"=w560:string)
                    n298 = Unbundle By Name(w567) -> ("WPSEL State"=w566:i32)
                    n299 = local read "WPSEL Status"() -> (w562:bool)
                    n300 = case shown="2" w566 {
                      tunnel: [cluster{u32, u32}[] [{9868950, 9868950}, {9868950, 9868950}] ("Colors [4]") cluster{u32, u32}[] [{9868950, 9868950}, {9868950, 9868950}] ("Colors [4]") cluster{u32, u32}[] [{16318208, 16318208}, {16318208, 16318208}] ("Colors [4]") cluster{u32, u32}[] [{6618880, 2424594}, {6618880, 2424594}] ("Colors [4]") w581] -> w565
                      tunnel: [FALSE ("WPROT Status") FALSE ("WPROT Status") TRUE ("WPROT Status") FALSE ("WPROT Status") w583] -> w564
                      tunnel: w562 -> [_ _ _ _ w582]
                      tunnel: ["" "" "" w577 ""] -> w561
                      tunnel: w560 -> [_ _ _ w577 _]
                      frame Default {
                      }
                      frame 0 {
                      }
                      frame 1 {
                      }
                      frame 2 {
                      }
                      frame 3 {
                        n301 = case shown="True" w582 {
                          tunnel: [cluster{u32, u32}[] [{7563008, 7563008}, {7563008, 7563008}] ("Colors [4]") cluster{u32, u32}[] [{16318208, 16318208}, {16318208, 16318208}] ("Colors [4]")] -> w581
                          frame False {
                          }
                          frame True {
                          }
                        }
                        n302 = Not(x=w582) -> (.not. x?=w583:bool)
                      }
                    }
                    "WPSEL Status" <- w564
                    "Waveplate" <- w564
                    n303 = property on="Waveplate" class="Bool (strict)"("Colors [4]"=w565, "BoolText.Text"=w561) -> ()  [unwired: 2 in, 2 out]
                    n304 = property on="WPSEL Status" class="Bool (strict)"("Colors [4]"=w565) -> ()  [unwired: 2 in, 2 out]
                  }
                  frame #1 {
                    # "WPROT"
                    n305 = Unbundle By Name(w589) -> ("WPROT State"=w588:i32)
                    n306 = case shown="2" w588 {
                      tunnel: [cluster{u32, u32}[] [{9868950, 9868950}, {9868950, 9868950}] ("Colors [4]") cluster{u32, u32}[] [{9868950, 9868950}, {9868950, 9868950}] ("Colors [4]") cluster{u32, u32}[] [{16318208, 16318208}, {16318208, 16318208}] ("Colors [4]") cluster{u32, u32}[] [{6618880, 6618880}, {6618880, 6618880}] ("Colors [4]") cluster{u32, u32}[] [{16318208, 16318208}, {16318208, 16318208}] ("Colors [4]")] -> w587
                      tunnel: [FALSE ("WPROT Status") FALSE ("WPROT Status") TRUE ("WPROT Status") FALSE ("WPROT Status") TRUE ("WPROT Status")] -> w586
                      frame Default {
                      }
                      frame 0 {
                      }
                      frame 1 {
                      }
                      frame 2 {
                      }
                      frame 3 {
                      }
                    }
                    "WPROT Status" <- w586
                    n307 = property on="WPROT Status" class="Bool (strict)"("Colors [4]"=w587) -> ()  [unwired: 2 in, 2 out]
                  }
                  frame #2 {
                    # "CALW"
                    n308 = Unbundle By Name(w607) -> ("CALW State"=w606:i32)
                    n309 = Unbundle By Name(w605) -> ("CALW posname"=w604:string)
                    n310 = local read "CALW Status"() -> (w600:bool)
                    n311 = case shown="3" w606 {
                      tunnel: [cluster{u32, u32}[] [{9868950, 9868950}, {9868950, 9868950}] ("Colors [4]") cluster{u32, u32}[] [{9868950, 9868950}, {9868950, 9868950}] ("Colors [4]") cluster{u32, u32}[] [{16318208, 16318208}, {16318208, 16318208}] ("Colors [4]") cluster{u32, u32}[] [{6618880, 6618880}, {6618880, 6618880}] ("Colors [4]") w627] -> w601
                      tunnel: [FALSE ("WPROT Status") FALSE ("WPROT Status") TRUE ("WPROT Status") FALSE ("WPROT Status") w629] -> w603
                      tunnel: w604 -> [_ _ _ w618 _]
                      tunnel: ["" "" "" w617 ""] -> w602
                      tunnel: w600 -> [_ _ _ _ w628]
                      frame Default {
                      }
                      frame 0 {
                      }
                      frame 1 {
                      }
                      frame 2 {
                        n312 = case shown="\"SHUTTER\"" w618 {
                          tunnel: ["" "DEPOL" "POL" "OFF" "PIN" "SHT"] -> w617
                          frame Default {
                          }
                          frame "DEPOLARIZER" {
                          }
                          frame "POLARIZER" {
